vi "ConvertFolderTDMS.vi"() -> ()   [LabVIEW 2017]
panel:
  in  "dossier destination":path
  out "sortie d'erreur":errorcluster
  out "chemin complet":path
  in  "chemin":path
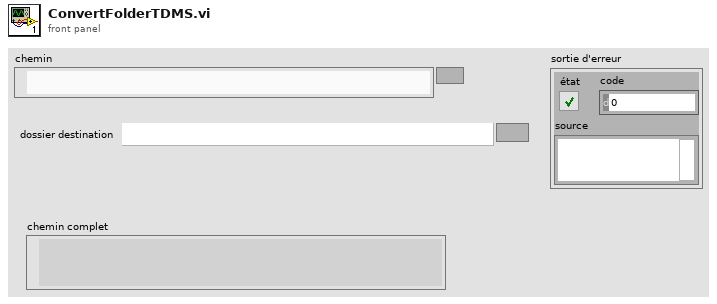
[diagram p1: front panel]
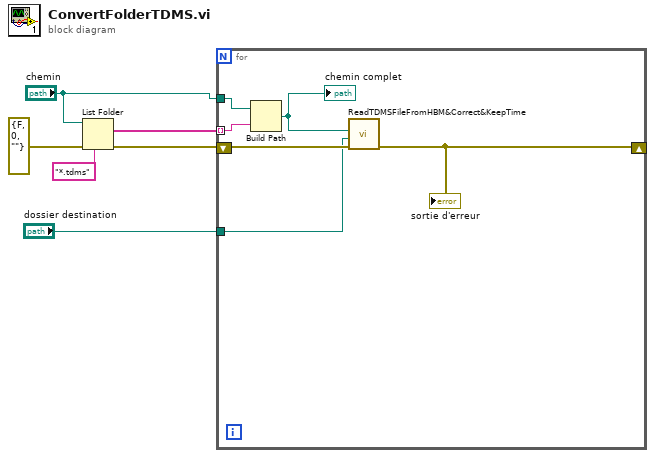
[diagram p0: block diagram]
diagram:
  n1 = List Folder(path="chemin", pattern="*.tdms" ("filtre"), error in=errorcluster {"status"=FALSE, "code"=0, "source"=""} ("entrée d'erreur")) -> (filenames=w5:string[], error out=w4:errorcluster)  [unwired: 1 in, 2 out]
  n2 = for {
    tunnel: w5 -> [w10] mode=indexing
    tunnel: "chemin" -> [w11]
    shift-right: [w8] -> _
    shift-left: w4 -> [w12]
    tunnel: "dossier destination" -> [w7]
    n3 = Build Path(base path=w11, name or relative path=w10) -> (appended path=w9:path)
    "chemin complet" <- w9
    n4 = call "ReadTDMSFileFromHBM&Correct&KeepTime.vi"("error in (no error)"=w12, "dossier destination"=w7, "file path"=w9) -> ("sortie d'erreur"=w8:errorcluster)  [unwired: 3 in, 1 out]
    "sortie d'erreur" <- w8
  }
